vi "fwInit.vi"(1 "FW init?":bool) -> (0 "Filter wheel init":cluster{"FW Handle":u32, "init?":i16})   [LabVIEW 2015]
panel:
  in  "FW current pos":u8 min=1 max=6
  in  "Device index":i32=3
  in  "Filter wheel":cluster{"FW Handle":u32, "init?":i16}
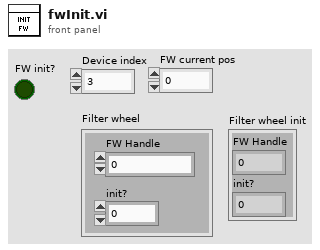
[diagram p1: front panel]
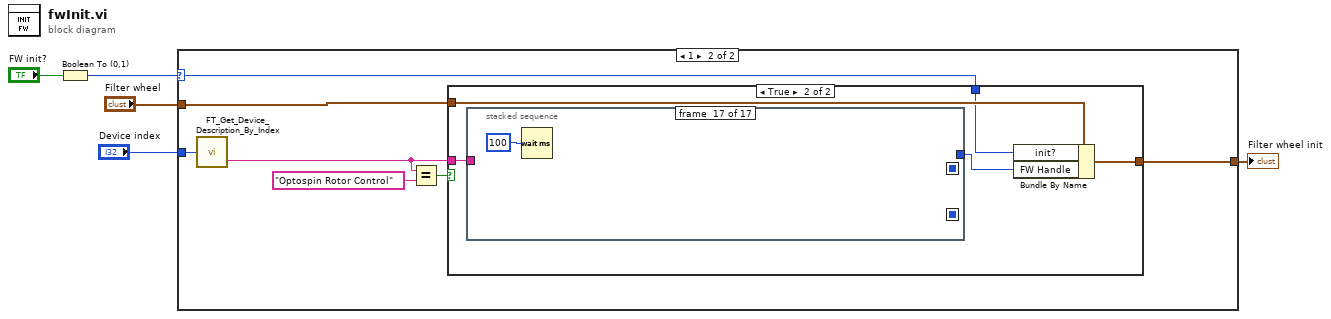
[diagram p0: block diagram]
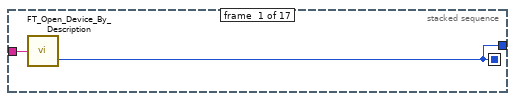
[diagram p4: hidden frame]
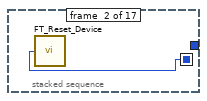
[diagram p5: hidden frame]
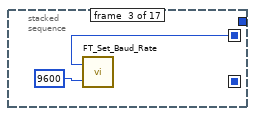
[diagram p6: hidden frame]
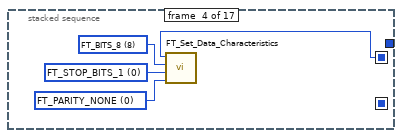
[diagram p7: hidden frame]
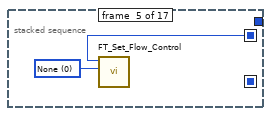
[diagram p8: hidden frame]
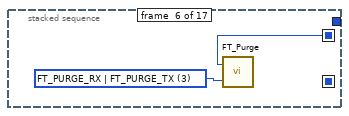
[diagram p9: hidden frame]
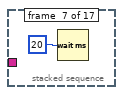
[diagram p10: hidden frame]
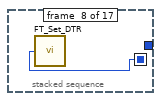
[diagram p11: hidden frame]
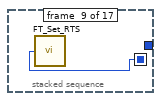
[diagram p12: hidden frame]
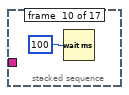
[diagram p13: hidden frame]
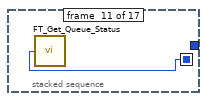
[diagram p14: hidden frame]
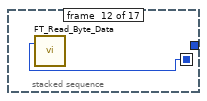
[diagram p15: hidden frame]
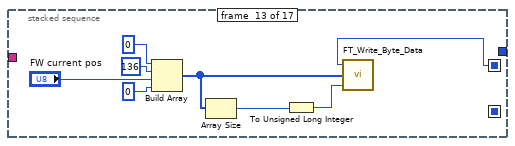
[diagram p16: hidden frame]
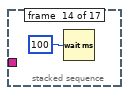
[diagram p17: hidden frame]
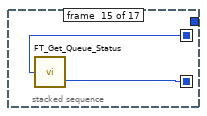
[diagram p18: hidden frame]
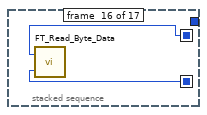
[diagram p19: hidden frame]
diagram:
  n1 = Boolean To (0,1)(Boolean="FW init?") -> (0, 1=w4:i16)
  n2 = case shown="1" w4 {
    selector: w4 -> [_ w7]
    tunnel: "Filter wheel" -> [_ w8]
    tunnel: "Device index" -> [_ w9]
    tunnel: [_ w6] -> w1
    frame 0, Default {
    }
    frame 1 {
      n3 = call "FT_Get_Device_Description_By_Index.vi"("Device Index"=w9) -> ("Device Description"=w10:string)  [unwired: 1 out]
      n4 = Equal?(x=w10, y="Optospin Rotor Control") -> (x = y?=w11:bool)
      n5 = case shown="True" w11 {
        tunnel: w10 -> [_ w17]
        tunnel: w8 -> [_ w16]
        tunnel: w7 -> [_ w15]
        tunnel: [_ w14] -> w6
        frame False {
        }
        frame True {
          n6 = stacked-sequence {
            seq-local: [w18 _ _ _ _ _ _ _ _ _ _ _ _ _ _ _ _] -> [_ w20 w21 w23 w27 w29 _ w32 w33 _ w35 w36 w37 _ w47 w49 _]
            seq-local: [_ _ _ _ _ _ _ _ _ _ _ _ _ _ w46 _ _] -> [_ _ _ _ _ _ _ _ _ _ _ _ _ _ _ w48 _]
            tunnel: w17 -> [w19 _ _ _ _ _ _ _ _ _ _ _ _ _ _ _ _]
            tunnel: [w18 _ _ _ _ _ _ _ _ _ _ _ _ _ _ _ _] -> w13
            frame #0 {
              n7 = call "FT_Open_Device_By_Description.vi"("Device Description"=w19) -> ("Handle"=w18:u32)  [unwired: 1 out]
            }
            frame #1 {
              n8 = call "FT_Reset_Device.vi"("Handle"=w20) -> ()  [unwired: 1 out]
            }
            frame #2 {
              n9 = call "FT_Set_Baud_Rate.vi"("Baud Rate"=u32 9600, "Handle"=w21) -> ()  [unwired: 1 out]
            }
            frame #3 {
              w24 = u8 0 items=["FT_PARITY_NONE", "FT_PARITY_ODD", "FT_PARITY_EVEN", "FT_PARITY_MARK", "FT_PARITY_SPACE"] ("Parity")
              w25 = u8 0 items=["FT_STOP_BITS_1"=0, "FT_STOP_BITS_2"=2] ("Stop Bits")
              w26 = u8 8 items=["FT_BITS_7"=7, "FT_BITS_8"=8] ("Word Length")
              n10 = call "FT_Set_Data_Characteristics.vi"("Parity"=w24, "Stop Bits"=w25, "Word Length"=w26, "Handle"=w23) -> ()  [unwired: 1 out]
            }
            frame #4 {
              w28 = u16 0 items=["None"=0, "RTS-CTS"=256, "DTR-DSR"=512, "XOn-XOff"=1024] ("Flow Control")
              n11 = call "FT_Set_Flow_Control.vi"("Flow Control"=w28, "Handle"=w27) -> ()  [unwired: 2 in, 1 out]
            }
            frame #5 {
              w30 = u32 3 items=["FT_PURGE_RX"=1, "FT_PURGE_TX"=2, "FT_PURGE_RX | FT_PURGE_TX"=3] ("Purge Flags")
              n12 = call "FT_Purge.vi"("Purge Flags"=w30, "Handle"=w29) -> ()  [unwired: 1 out]
            }
            frame #6 {
              n13 = Wait (ms)(milliseconds to wait=u32 20) -> ()  [unwired: 1 out]
            }
            frame #7 {
              n14 = call "FT_Set_DTR.vi"("Handle"=w32) -> ()  [unwired: 1 out]
            }
            frame #8 {
              n15 = call "FT_Set_RTS.vi"("Handle"=w33) -> ()  [unwired: 1 out]
            }
            frame #9 {
              n16 = Wait (ms)(milliseconds to wait=u32 100) -> ()  [unwired: 1 out]
            }
            frame #10 {
              n17 = call "FT_Get_Queue_Status.vi"("Handle"=w35) -> ()  [unwired: 2 out]
            }
            frame #11 {
              n18 = call "FT_Read_Byte_Data.vi"("Handle"=w36) -> ()  [unwired: 1 in, 3 out]
            }
            frame #12 {
              n19 = Build Array(u8 0 ("element"), u8 136 ("element"), "FW current pos", u8 0 ("element")) -> (w38:u8[])
              n20 = Array Size(array=w38) -> (size(s)=w40:i32)
              n21 = To Unsigned Long Integer(number=w40) -> (unsigned 32bit integer=w39:u32)
              n22 = call "FT_Write_Byte_Data.vi"("Bytes To Write"=w39, "Buffer"=w38, "Handle"=w37) -> ()  [unwired: 2 out]
            }
            frame #13 {
              n23 = Wait (ms)(milliseconds to wait=u32 100) -> ()  [unwired: 1 out]
            }
            frame #14 {
              n24 = call "FT_Get_Queue_Status.vi"("Handle"=w47) -> ("Bytes Waiting"=w46:u32)  [unwired: 1 out]
            }
            frame #15 {
              n25 = call "FT_Read_Byte_Data.vi"("Handle"=w49, "Bytes To Read"=w48) -> ()  [unwired: 3 out]
            }
            frame #16 {
              n26 = Wait (ms)(milliseconds to wait=u32 100) -> ()  [unwired: 1 out]
            }
          }
          n27 = Bundle By Name(cluster=w16, "init?"=w15, "FW Handle"=w13) -> (w14:cluster{"FW Handle":u32, "init?":i16})
        }
      }
    }
  }
  "Filter wheel init" <- w1
